vi "Gears.vi"   [LabVIEW 2016]
uses:
  <vilib>/Rock Robotics/WPI/Solenoid/WPI_SolenoidValue.ctl
  <vilib>/Rock Robotics/WPI/Solenoid/WPI_SolenoidSetEnum.vi
  <vilib>/Rock Robotics/WPI/Utilities/WPI_GetSetVariantRefNum.vi
types:
  T1 = typedef "WPI_DriverStationRobotMode2.ctl" = enum16{"Autonomous Disabled", "Autonomous Enabled", "Teleop Disabled", "Teleop Enabled", "Disconnected", "Finish", "Test Disabled", "Test Enabled", "Emergency Stopped"}
  T2 = typedef "WPI_SolenoidValue.ctl" = enum16{"Off", "On", "Forward", "Reverse"}
  T3 = typedef "WPI_SolenoidDevRef.ctl" = cluster{"DevStatus":errorcluster, "Pneumatics Control Module":u8, "Forward Solenoid Channel":T4, "Reverse Solenoid Channel":T4}
  T4 = typedef "WPI_SolenoidChannel.ctl" = enum8{"Solenoid 0", "Solenoid 1", "Solenoid 2", "Solenoid 3", "Solenoid 4", "Solenoid 5", "Solenoid 6", "Solenoid 7", "Invalid"}
  T5 = typedef "WPI_JoystickDevRef.ctl" = cluster{"Device":T6}
  T6 = typedef "WPI_JoystickDeviceEnum.ctl" = enum16{"USB 0", "USB 1", "USB 2", "USB 3", "USB 4", "USB 5"}
  T7 = typedef "WPI_DigitalInputDevRef.ctl" = cluster{"DevStatus":errorcluster, "DIO Channel":T8}
  T8 = typedef "FPGA_DIOChannel.ctl" = enum8{"DIO 0", "DIO 1", "DIO 2", "DIO 3", "DIO 4", "DIO 5", "DIO 6", "DIO 7", "DIO 8", "DIO 9", "DIO MXP 0", "DIO MXP 1", "DIO MXP 2", "DIO MXP 3", "DIO MXP 4", "DIO MXP 5", "DIO MXP 6", "DIO MXP 7", "DIO MXP 8", "DIO MXP 9", "DIO MXP 10", "DIO MXP 11", "DIO MXP 12", "DIO MXP 13", "DIO MXP 14", "DIO MXP 15", "SPI Port CS1", "SPI Port CS2", "SPI Port CS3", "SPI Port MISO", "SPI Port MOSI", "Invalid"}
  T9 = typedef "WPI_MotorControlDeviceRef.ctl" = cluster{"DeviceStatus":errorcluster, "Type":T10, "PWM":cluster{"PWM Channel":T11, "DeadBand":T12}, "CAN":cluster{"Device Number":u8, "SetOutput VI Ref":variant, "GetOutput VI Ref":variant, "Enable VI Ref":variant, "Disable VI Ref":variant, "Data":variant}, "Invert":bool}
  T10 = typedef "WPI_MotorControlType.ctl" = enum16{"PWM", "CAN"}
  T11 = typedef "FPGA_DIOPWMChannel.ctl" = enum8{"PWM 0", "PWM 1", "PWM 2", "PWM 3", "PWM 4", "PWM 5", "PWM 6", "PWM 7", "PWM 8", "PWM 9", "PWM MXP 0", "PWM MXP 1", "PWM MXP 2", "PWM MXP 3", "PWM MXP 4", "PWM MXP 5", "PWM MXP 6", "PWM MXP 7", "PWM MXP 8", "PWM MXP 9", "Invalid"}
  T12 = typedef "WPI_PWMDeadband.ctl" = cluster{"Name":string, "maxPositivePwm":i32, "minPositivePwm":i32, "centerPwm":i32, "maxNegativePwm":i32, "minNegativePwm":i32, "angularRange":u16}
  T13 = typedef "WPI_ServoDeviceRef.ctl" = cluster{"DeviceStatus":errorcluster, "PWM Channel":T11, "DeadBand":T12}
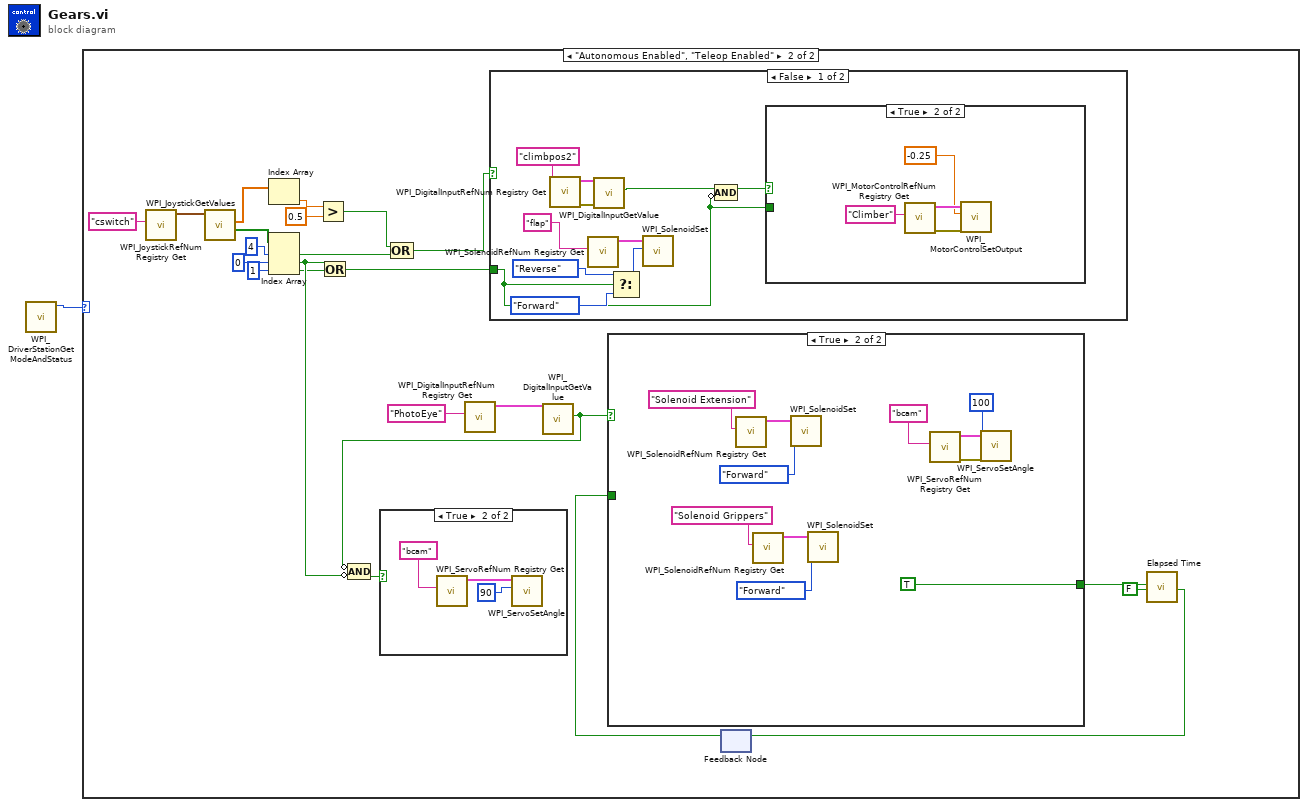
[diagram p0: block diagram]
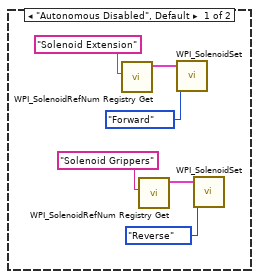
[diagram p2: hidden frame]
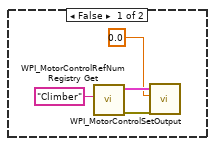
[diagram p4: hidden frame]
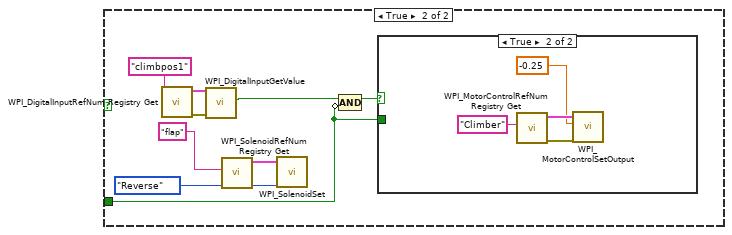
[diagram p5: hidden frame]
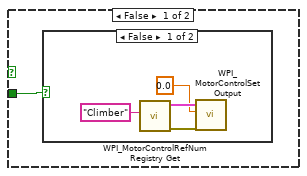
[diagram p6: hidden frame]
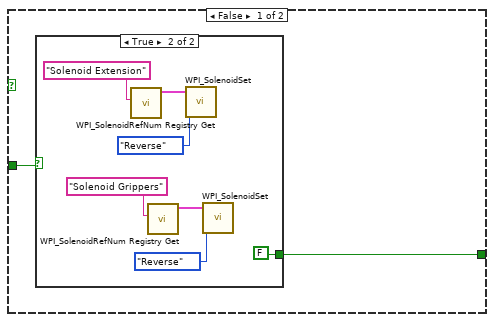
[diagram p9: hidden frame]
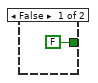
[diagram p10: hidden frame]
diagram:
  n1 = call <vilib>:"WPI_DriverStationGetModeAndStatus.vi"() -> ("Robot Mode"=w1:T1)  [unwired: 10 in, 1 out]
  n2 = case shown="\"Autonomous Enabled\", \"Teleop Enabled\"" w1 {
    frame "Autonomous Disabled", Default {
      n3 = call <vilib>:"WPI_SolenoidRefNum Registry Get.vi"("refnum name"="Solenoid Extension") -> ("SolenoidDevRef"=w3:T3)  [unwired: 9 in, 1 out]
      n4 = call <vilib>:"WPI_SolenoidRefNum Registry Get.vi"("refnum name"="Solenoid Grippers") -> ("SolenoidDevRef"=w7:T3)  [unwired: 9 in, 1 out]
      n5 = call-poly <vilib>:"WPI_SolenoidSet.vi"("Value"=WPI_SolenoidValue."Forward", "SolenoidDevRef"=w3) -> ()  [unwired: 8 in, 2 out]
      n6 = call-poly <vilib>:"WPI_SolenoidSet.vi"("Value"=WPI_SolenoidValue."Reverse", "SolenoidDevRef"=w7) -> ()  [unwired: 8 in, 2 out]
    }
    frame "Autonomous Enabled", "Teleop Enabled" {
      n7 = call <vilib>:"WPI_JoystickRefNum Registry Get.vi"("refnum name"="cswitch") -> ("JoystickDevRef"=w20:T5)  [unwired: 9 in, 1 out]
      n8 = call <vilib>:"WPI_JoystickGetValues.vi"("JoystickDevRef"=w20) -> ("Buttons"=w23:bool[], "Axes"=w13:dbl[])  [unwired: 6 in, 3 out]
      n9 = Index Array(array=w13) -> (element=w11:dbl)  [unwired: 1 in]
      n10 = Index Array(array=w23, index #1=4 ("index"), index #2=0 ("index"), index #3=1 ("index")) -> (element #1=w14:bool, element #2=w17:bool, element #3=w16:bool)
      n11 = Greater?(x=w11, y=0.5) -> (0:w9:bool)
      n12 = Or(x=w17, y=w16) -> (x .or. y?=w15:bool)
      n13 = Compound Arithmetic op=OR(w9, w14) -> (w12:bool)
      n14 = call <vilib>:"WPI_DigitalInputRefNum Registry Get.vi"("refnum name"="PhotoEye") -> ("DigitalInputDevRef"=w29:T7)  [unwired: 9 in, 1 out]
      n15 = case shown="False" w12 {
        tunnel: w15 -> [w32 w52]
        frame False {
          n16 = call <vilib>:"WPI_DigitalInputRefNum Registry Get.vi"("refnum name"="climbpos2") -> ("error out"=w41:errorcluster, "DigitalInputDevRef"=w40:T7)  [unwired: 9 in]
          n17 = call <vilib>:"WPI_SolenoidRefNum Registry Get.vi"("refnum name"="flap") -> ("SolenoidDevRef"=w36:T3)  [unwired: 9 in, 1 out]
          n18 = call <vilib>:"WPI_DigitalInputGetValue.vi"("error in (no error)"=w41, "DigitalInputDevRef"=w40) -> ("Value"=w38:bool)  [unwired: 7 in, 2 out]
          n19 = Select(t=WPI_SolenoidValue."Reverse" ("Value"), s=w32, f=WPI_SolenoidValue."Forward" ("Value")) -> (s? t:f=w31:T2)
          n20 = call-poly <vilib>:"WPI_SolenoidSet.vi"("Value"=w31, "SolenoidDevRef"=w36) -> ()  [unwired: 8 in, 2 out]
          n21 = Compound Arithmetic op=AND(w38, invert w32) -> (w35:bool)
          n22 = case shown="True" w35 {
            tunnel: w32 -> [w42 _]
            frame False {
              n23 = case shown="True" w42 {
                frame False {
                  n24 = call <vilib>:"WPI_MotorControlRefNum Registry Get.vi"("refnum name"="Climber") -> ("error out"=w45:errorcluster, "MotorControlDevRef"=w46:T9)  [unwired: 9 in]
                  n25 = call <vilib>:"WPI_MotorControlSetOutput.vi"("error in (no error)"=w45, "Output"=0.0, "MotorControlDevRef"=w46) -> ()  [unwired: 6 in, 3 out]
                }
                frame True {
                }
              }
            }
            frame True {
              n26 = call <vilib>:"WPI_MotorControlRefNum Registry Get.vi"("refnum name"="Climber") -> ("error out"=w49:errorcluster, "MotorControlDevRef"=w50:T9)  [unwired: 9 in]
              n27 = call <vilib>:"WPI_MotorControlSetOutput.vi"("error in (no error)"=w49, "Output"=-0.25, "MotorControlDevRef"=w50) -> ()  [unwired: 6 in, 3 out]
            }
          }
        }
        frame True {
          n28 = call <vilib>:"WPI_DigitalInputRefNum Registry Get.vi"("refnum name"="climbpos1") -> ("error out"=w57:errorcluster, "DigitalInputDevRef"=w56:T7)  [unwired: 9 in]
          n29 = call <vilib>:"WPI_DigitalInputGetValue.vi"("error in (no error)"=w57, "DigitalInputDevRef"=w56) -> ("Value"=w54:bool)  [unwired: 7 in, 2 out]
          n30 = call <vilib>:"WPI_SolenoidRefNum Registry Get.vi"("refnum name"="flap") -> ("SolenoidDevRef"=w59:T3)  [unwired: 9 in, 1 out]
          n31 = call-poly <vilib>:"WPI_SolenoidSet.vi"("Value"=WPI_SolenoidValue."Reverse", "SolenoidDevRef"=w59) -> ()  [unwired: 8 in, 2 out]
          n32 = Compound Arithmetic op=AND(w54, invert w52) -> (w53:bool)
          n33 = case shown="True" w53 {
            tunnel: w52 -> [w60 _]
            frame False {
              n34 = case shown="False" w60 {
                frame False {
                  n35 = call <vilib>:"WPI_MotorControlRefNum Registry Get.vi"("refnum name"="Climber") -> ("error out"=w63:errorcluster, "MotorControlDevRef"=w64:T9)  [unwired: 9 in]
                  n36 = call <vilib>:"WPI_MotorControlSetOutput.vi"("error in (no error)"=w63, "Output"=0.0, "MotorControlDevRef"=w64) -> ()  [unwired: 6 in, 3 out]
                }
                frame True {
                }
              }
            }
            frame True {
              n37 = call <vilib>:"WPI_MotorControlRefNum Registry Get.vi"("refnum name"="Climber") -> ("error out"=w67:errorcluster, "MotorControlDevRef"=w68:T9)  [unwired: 9 in]
              n38 = call <vilib>:"WPI_MotorControlSetOutput.vi"("error in (no error)"=w67, "Output"=-0.25, "MotorControlDevRef"=w68) -> ()  [unwired: 6 in, 3 out]
            }
          }
        }
      }
      n39 = call <vilib>:"WPI_DigitalInputGetValue.vi"("DigitalInputDevRef"=w29) -> ("Value"=w25:bool)  [unwired: 8 in, 2 out]
      n40 = Compound Arithmetic op=AND(invert w25, invert w17) -> (w24:bool)
      n41 = case shown="True" w24 {
        frame False {
        }
        frame True {
          n42 = call <vilib>:"WPI_ServoRefNum Registry Get.vi"("refnum name"="bcam") -> ("ServoDeviceRef"=w70:T13)  [unwired: 9 in, 1 out]
          n43 = call <vilib>:"WPI_ServoSetAngle.vi"("Angle"=90, "ServoDeviceRef"=w70) -> ()  [unwired: 8 in, 2 out]
        }
      }
      n44 = feedback #1() -> (w26:bool)  [unwired: 1 in]
      n45 = case shown="True" w25 {
        tunnel: [w72 TRUE] -> w28
        tunnel: w26 -> [w73 _]
        frame False {
          n46 = case shown="True" w73 {
            tunnel: [FALSE FALSE] -> w72
            frame False {
            }
            frame True {
              n47 = call <vilib>:"WPI_SolenoidRefNum Registry Get.vi"("refnum name"="Solenoid Extension") -> ("SolenoidDevRef"=w77:T3)  [unwired: 9 in, 1 out]
              n48 = call <vilib>:"WPI_SolenoidRefNum Registry Get.vi"("refnum name"="Solenoid Grippers") -> ("SolenoidDevRef"=w81:T3)  [unwired: 9 in, 1 out]
              n49 = call-poly <vilib>:"WPI_SolenoidSet.vi"("Value"=WPI_SolenoidValue."Reverse", "SolenoidDevRef"=w77) -> ()  [unwired: 8 in, 2 out]
              n50 = call-poly <vilib>:"WPI_SolenoidSet.vi"("Value"=WPI_SolenoidValue."Reverse", "SolenoidDevRef"=w81) -> ()  [unwired: 8 in, 2 out]
            }
          }
        }
        frame True {
          n51 = call <vilib>:"WPI_SolenoidRefNum Registry Get.vi"("refnum name"="Solenoid Extension") -> ("SolenoidDevRef"=w83:T3)  [unwired: 9 in, 1 out]
          n52 = call <vilib>:"WPI_SolenoidRefNum Registry Get.vi"("refnum name"="Solenoid Grippers") -> ("SolenoidDevRef"=w87:T3)  [unwired: 9 in, 1 out]
          n53 = call-poly <vilib>:"WPI_SolenoidSet.vi"("Value"=WPI_SolenoidValue."Forward", "SolenoidDevRef"=w83) -> ()  [unwired: 8 in, 2 out]
          n54 = call-poly <vilib>:"WPI_SolenoidSet.vi"("Value"=WPI_SolenoidValue."Forward", "SolenoidDevRef"=w87) -> ()  [unwired: 8 in, 2 out]
          n55 = call <vilib>:"WPI_ServoRefNum Registry Get.vi"("refnum name"="bcam") -> ("error out"=w90:errorcluster, "ServoDeviceRef"=w89:T13)  [unwired: 9 in]
          n56 = call <vilib>:"WPI_ServoSetAngle.vi"("error in (no error)"=w90, "Angle"=100, "ServoDeviceRef"=w89) -> ()  [unwired: 7 in, 2 out]
        }
      }
      n57 = call "Elapsed Time"("Reset"=w28, "Auto Reset"=FALSE) -> ("Time has Elapsed"=w27:bool)  [unwired: 10 in, 7 out]
      n58 = feedback-in #1(w27) -> ()
    }
  }
